vi "Datasheet Build Array of Plot-Run.vi"(4 "System or ALL Combined Fields":T1[](array[typedef]), 8 "error in (no error)":errorcluster, 9 "Connection Refnum":T4, 10 "Parameters":T5, 11 "Result Group":T9[](array[typedef])) -> (0 "error out":errorcluster, 1 "Connection Refnum":T4, 2 "Updated Parameter":T5, 3 "Runs for Each Plot":T6[][](array[typedef]))   [LabVIEW 2011]
uses:
  TDMS/TDMS File.ctl
  TDMS/TDMS Run.ctl
  TDMS/TDMS Channel (Sxx).ctl
  database/Fields/Field Record.ctl
  database/Fields/Field DataTypes.ctl
  database/Fields/Field NextItem.ctl
  Addons/internet/utils/keyedarr.llb/Keyed Array.ctl
  www/cgi-bin/_cgi-lib/TDM_INDEX Record.ctl
  SI.LIB/ODBC/SQL Controls/Connection Refnum.ctl
  Addons/internet/utils/strutil.llb/Case Matching.ctl
panel:
  in  "File Information":T6
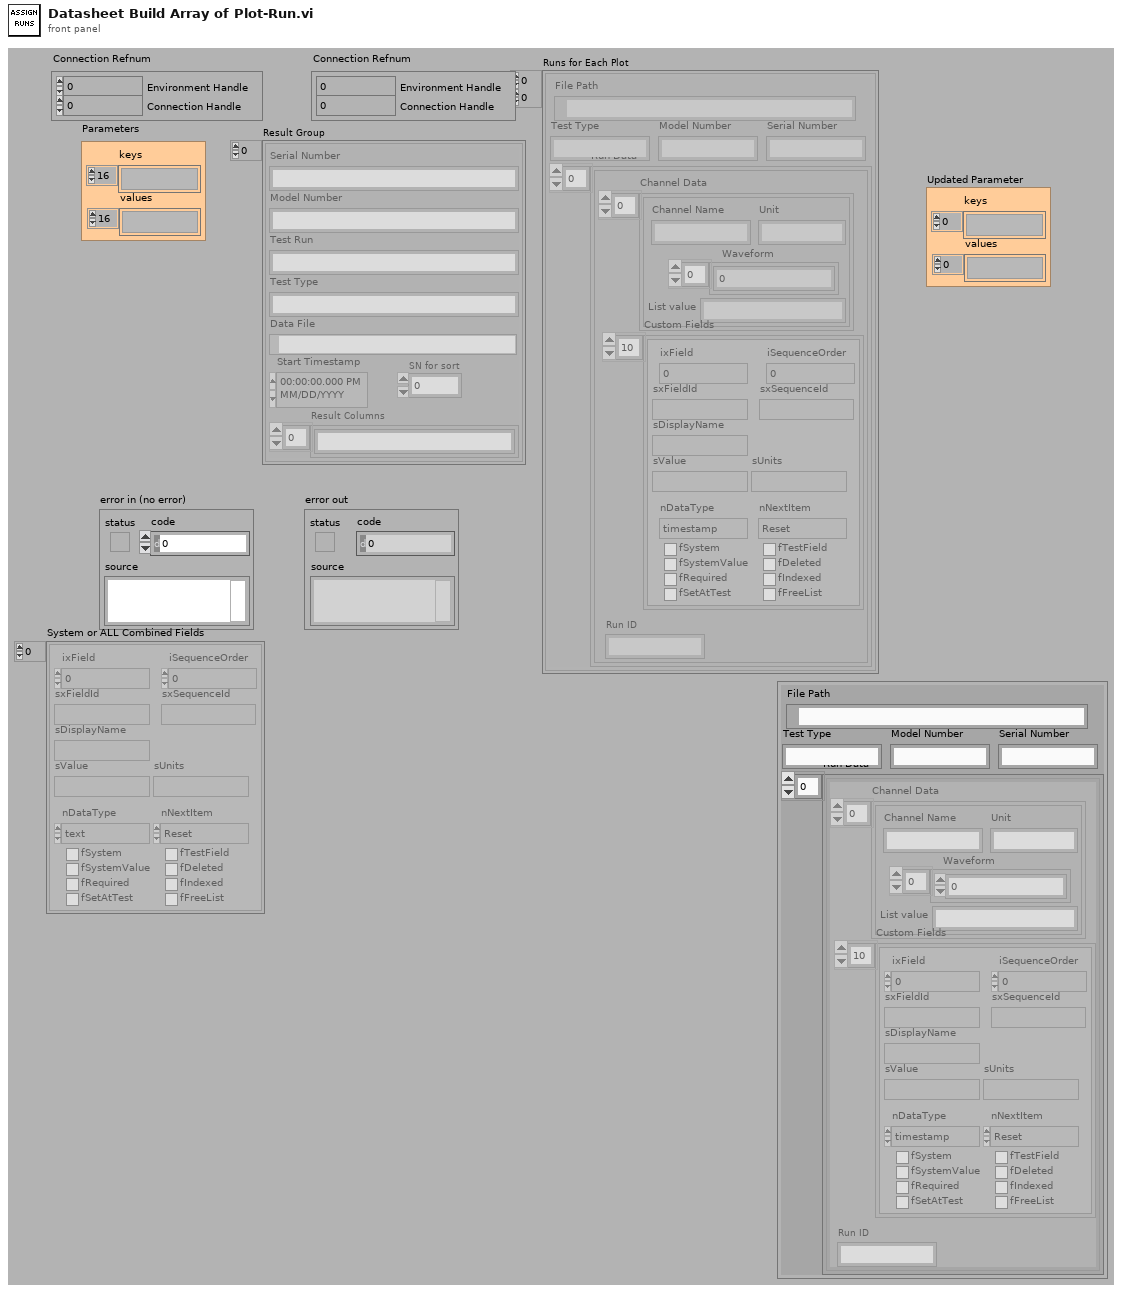
[diagram p1: front panel]
types:
  T1 = typedef "Field Record.ctl" = cluster{"ixField":i32, "iSequenceOrder":i32, "sxFieldId":string, "sxSequenceId":string, "sDisplayName":string, "sValue":string, "sUnits":string, "nDataType":T2, "nNextItem":T3, "fSystem":bool, "fSystemValue":bool, "fRequired":bool, "fSetAtTest":bool, "fTestField":bool, "fDeleted":bool, "fIndexed":bool, "fFreeList":bool}
  T2 = typedef "Field DataTypes.ctl" = enum32{"text", "numeric", "list", "timestamp", "boolean"}
  T3 = typedef "Field NextItem.ctl" = enum32{"Reset", "Retain", "Auto-Increment"}
  T4 = typedef "Connection Refnum.ctl" = cluster{"Environment Handle":i32, "Connection Handle":i32}
  T5 = typedef "Keyed Array.ctl" = cluster{"keys":string[], "values":string[]}
  T6 = typedef "TDMS File.ctl" = cluster{"File Path":path, "Run Data":T7[], "Serial Number":string, "Model Number":string, "Test Type":string}
  T7 = typedef "TDMS Run.ctl" = cluster{"Channel Data":T8[], "Custom Fields":T1[], "Run ID":string}
  T8 = typedef "TDMS Channel (Sxx).ctl" = cluster{"Channel Name":string, "Waveform":dbl[], "Unit":string, "List value":string}
  T9 = typedef "TDM_INDEX Record.ctl" = cluster{"Model Number":string, "SN for sort":i32, "Test Type":string, "Test Run":string, "Serial Number":string, "Start Timestamp":timestamp, "Data File":path, "Result Columns":string[]}
  T10 = typedef "Case Matching.ctl" = enum16{"a != A", "a == A", "system"}
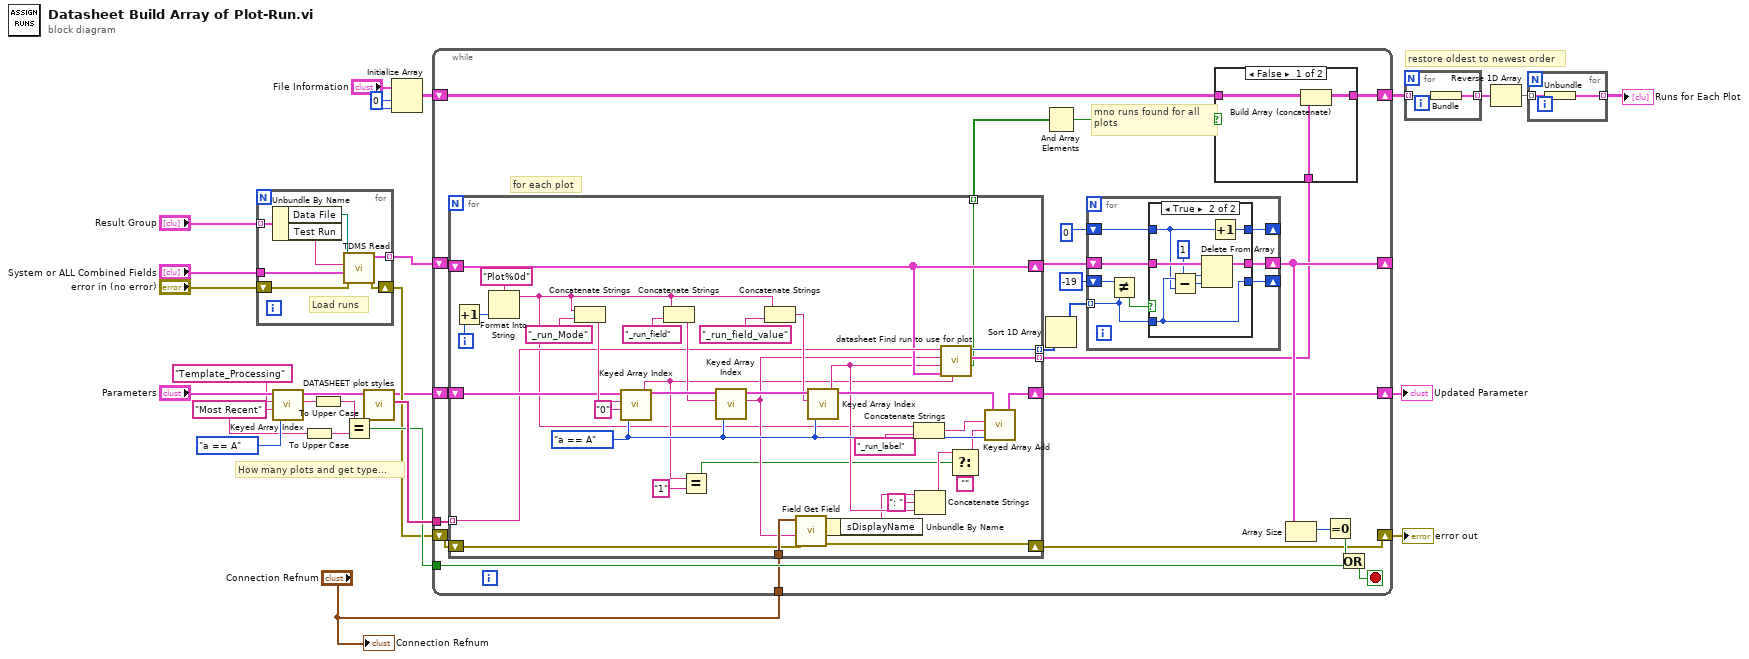
[diagram p0: block diagram]
diagram:
  w12 = 0 ("dimension size")
  w18 = "Most Recent" ("default value")
  # "restore oldest to newest order"
  # "How many plots and get type..."
  n1 = for {
    tunnel: "Result Group" -> [w32] mode=indexing
    shift-right: [w31] -> w6
    shift-left: "error in (no error)" -> [w28]
    tunnel: [w30] -> w20 mode=indexing
    tunnel: "System or ALL Combined Fields" -> [w29]
    # "Load runs"
    n2 = Unbundle By Name(w32) -> ("Data File"=w27:path, "Test Run"=w33:string)
    n3 = call "TDMS Read.vi"("error in (no error)"=w28, "System or ALL Combined Fields"=w29, "Run String"=w33, "TDM File Path"=w27) -> ("error out"=w31:errorcluster, "File Information"=w30:T6)  [unwired: 3 in, 3 out]
  }
  n4 = call "Keyed Array Index.vi"("case matching (sensitive)"=Case_Matching."a == A", "default value"=w18, "key"="Template_Processing" ("default value"), "array in"="Parameters") -> ("value"=w19:string, "duplicate array"=w21:T5)  [unwired: 2 out]
  n5 = To Upper Case(1:w18) -> (0:w17:string)
  n6 = To Upper Case(1:w19) -> (0:w16:string)
  n7 = Equal?(x=w16, y=w17) -> (x = y?=w15:bool)
  n8 = call "DATASHEET plot styles.vi"("parameters"=w21) -> ("styles"=w22:string[], "parameters 2"=w1:T5)  [unwired: 9 in]
  n9 = Initialize Array("File Information", w12, w12) -> (w13:T6[][])
  n10 = while {
    tunnel: w22 -> [w55]
    shift-right: [w47] -> _
    shift-left: w20 -> [w53]
    tunnel: w15 -> [w43]
    shift-right: [w39] -> w11
    shift-left: w13 -> [w40]
    shift-right: [w37] -> w7
    shift-left: w1 -> [w54]
    shift-right: [w35] -> w5
    shift-left: w6 -> [w36]
    tunnel: "Connection Refnum" -> [w34]
    stop <- w44 stop-if-true
    # "mno runs found for all \nplots"
    # "for each plot"
    n11 = for {
      tunnel: w55 -> [w102] mode=indexing
      shift-right: [w100] -> w51
      shift-left: w53 -> [w100]
      tunnel: [w101] -> w38 mode=indexing
      tunnel: [w99] -> w52 mode=indexing
      tunnel: [w98] -> w42 mode=indexing
      shift-right: [w95] -> w37
      shift-left: w54 -> [w103]
      shift-right: [w90] -> w35
      shift-left: w36 -> [w91]
      tunnel: w34 -> [w92]
      i -> [w104]
      w93 = Case_Matching."a == A" ("case matching (sensitive)")
      n12 = Increment(x=w104) -> (x+1=w113:i32)
      n13 = Format Into String(format string="Plot%0d", w113) -> (resulting string=w78:string)  [unwired: 2 in, 1 out]
      n14 = Concatenate Strings(w78, "_run_Mode" ("format string")) -> (w109:string)
      n15 = call "Keyed Array Index.vi"("case matching (sensitive)"=w93, "default value"="0", "key"=w109, "array in"=w103) -> ("value"=w84:string, "duplicate array"=w108:T5)  [unwired: 2 out]
      n16 = Concatenate Strings(w78, "_run_field" ("format string")) -> (w105:string)
      n17 = Equal?(x=w84, y="1") -> (x = y?=w81:bool)
      n18 = call "Keyed Array Index.vi"("case matching (sensitive)"=w93, "key"=w105, "array in"=w108) -> ("value"=w89:string, "duplicate array"=w107:T5)  [unwired: 1 in, 2 out]
      n19 = Concatenate Strings(w78, "_run_field_value" ("format string")) -> (w106:string)
      n20 = call "Field Get Field.vi"("error in (no error)"=w91, "sFieldId or sDisplayName (\"\")"=w89, "Connection Refnum"=w92) -> ("error out"=w90:errorcluster, "Field"=w88:T1)  [unwired: 2 in, 5 out]
      n21 = call "Keyed Array Index.vi"("case matching (sensitive)"=w93, "key"=w106, "array in"=w107) -> ("value"=w87:string, "duplicate array"=w96:T5)  [unwired: 1 in, 2 out]
      n22 = Unbundle By Name(w88) -> ("sDisplayName"=w86:string)
      n23 = Concatenate Strings(w78, "_run_label" ("format string")) -> (w94:string)
      n24 = Concatenate Strings(w86, ": " ("string"), w87) -> (w82:string)
      n25 = call "datasheet Find run to use for plot.vi"("Run Mode"=w84, "run array"=w100, "Field Value"=w87, "Field"=w89, "Test Type"=w102) -> ("no runs found"=w98:bool, "Run to Use"=w101:T6, "run used"=w99:i32)  [unwired: 2 in, 2 out]
      n26 = Select(t=w82, s=w81, f="") -> (s? t:f=w80:string)
      n27 = call "Keyed Array Add.vi"("case matching (sensitive)"=w93, "value"=w80, "key"=w94, "array in"=w96) -> ("array out"=w95:T5)  [unwired: 3 out]
    }
    n28 = And Array Elements(Boolean array=w42) -> (logical AND=w41:bool)
    n29 = Sort 1D Array(array=w52) -> (sorted array=w49:i32[])
    n30 = for {
      shift-right: [w66] -> w47
      shift-left: w51 -> [w67]
      shift-right: [w60] -> _
      shift-left: -19 -> [w65]
      tunnel: w49 -> [w61] mode=indexing
      shift-right: [w62] -> _
      shift-left: 0 -> [w63]
      n31 = Not Equal?(x=w65, y=w61) -> (x != y?=w64:bool)
      n32 = case shown="True" w64 {
        tunnel: w67 -> [w70 w77]
        tunnel: [w70 w76] -> w66
        tunnel: w63 -> [w69 w73]
        tunnel: [w69 w75] -> w62
        tunnel: w61 -> [w68 w74]
        tunnel: [w68 w74] -> w60
        frame False {
          # "already\ndeleted"
        }
        frame True {
          n33 = Subtract(x=w74, y=w73) -> (x-y=w71:i32)
          n34 = Delete From Array(array=w77, length=1, index=w71) -> (array with subset deleted=w76:T6[])  [unwired: 1 out]
          n35 = Increment(x=w73) -> (x+1=w75:i32)
        }
      }
    }
    n36 = case shown="False" w41 {
      tunnel: w40 -> [w58 w59]
      tunnel: [w57 w59] -> w39
      tunnel: w38 -> [w56 _]
      frame False {
        n37 = Build Array (concatenate)(w58, w56) -> (w57:T6[][])
      }
      frame True {
      }
    }
    n38 = Array Size(array=w47) -> (size(s)=w46:i32)
    n39 = Equal To 0?(x=w46) -> (x = 0?=w45:bool)
    n40 = Or(x=w45, y=w43) -> (x .or. y?=w44:bool)
  }
  "Updated Parameter" <- w7
  "error out" <- w5
  n41 = for {
    tunnel: w11 -> [w117] mode=indexing
    tunnel: [w116] -> w10 mode=indexing
    n42 = Bundle(w117) -> (w116:cluster{T6[]})  [unwired: 1 in]
  }
  n43 = Reverse 1D Array(array=w10) -> (reversed array=w8:cluster{T6[]}[])
  n44 = for {
    tunnel: w8 -> [w119] mode=indexing
    tunnel: [w118] -> w9 mode=indexing
    n45 = Unbundle(w119) -> (w118:T6[])
  }
  "Runs for Each Plot" <- w9
  "Connection Refnum" <- "Connection Refnum"
